vi "CT_TriggerDataAcq.vi"(6 "milliseconds to wait":u32=30, 8 "Error In":errorcluster caption="error out", 11 "Trigger Channel":refnum<k21>="PCIe-VF_MeasureTrigCu1") -> (0 "Error Out":errorcluster caption="error out")   [LabVIEW 2016]
uses:
  <vilib>/DAQmx/write.llb/DAQmx Write (Digital Bool 1Line 1Point).vi
  <vilib>/DAQmx/miscellaneous.llb/DAQmx Fill In Error Info.vi
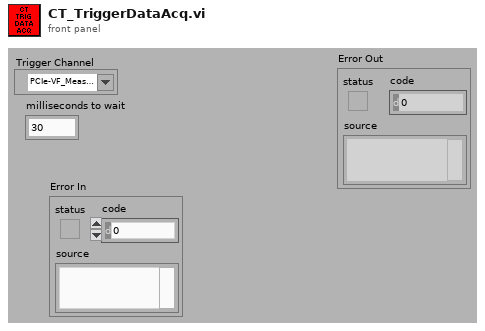
[diagram p1: front panel]
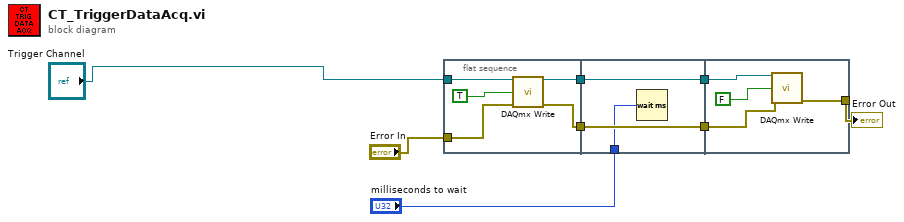
[diagram p0: block diagram]
diagram:
  n1 = flat-sequence {
    tunnel: "Trigger Channel" -> [w12]
    tunnel: [w11] -> w8
    tunnel: "Error In" -> [w10]
    tunnel: [w9] -> w4
    tunnel: [w16] -> w7
    tunnel: w8 -> [w16]
    tunnel: [w15] -> w5
    tunnel: w4 -> [w15]
    tunnel: "milliseconds to wait" -> [w14]
    tunnel: w7 -> [w20]
    tunnel: w5 -> [w18]
    tunnel: [w17] -> w3
    frame #0 {
      n2 = call-poly <vilib>:"DAQmx Write.vi"("task/channels in"=w12, "data"=TRUE, "error in"=w10) -> ("task out"=w11:refnum<k21>, "error out"=w9:errorcluster)  [unwired: 10 in, 1 out]
    }
    frame #1 {
      n3 = Wait (ms)(milliseconds to wait=w14) -> ()  [unwired: 1 out]
    }
    frame #2 {
      n4 = call-poly <vilib>:"DAQmx Write.vi"("task/channels in"=w20, "data"=FALSE, "error in"=w18) -> ("error out"=w17:errorcluster)  [unwired: 10 in, 2 out]
    }
  }
  "Error Out" <- w3
